vi "IMAQDevice.contents.vi"() -> ()   [LabVIEW 2014, in "IMAQDevice.lvlib"]
uses:
  IMAQDevice.lvlib
panel:
  out "error out":errorcluster
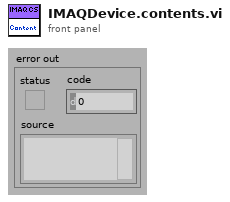
[diagram p1: front panel]
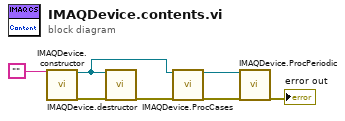
[diagram p0: block diagram]
diagram:
  n1 = call "IMAQDevice.constructor.vi"("name"="") -> ("i ref out"=w6:refnum<vi>, "error out"=w7:errorcluster)  [unwired: 16 in, 1 out]
  n2 = call "IMAQDevice.destructor.vi"("i ref in"=w6, "error in (no error)"=w7) -> ("error out"=w3:errorcluster)  [unwired: 17 in]
  n3 = call "IMAQDevice.ProcCases.vi"("i ref in"=w6, "error in (no error)"=w3) -> ("i ref out"=w5:refnum<vi>, "error out"=w4:errorcluster)  [unwired: 15 in, 1 out]
  n4 = call "IMAQDevice.ProcPeriodic.vi"("i ref in"=w5, "error in (no error)"=w4) -> ("error out"=→"error out":errorcluster)  [unwired: 15 in, 2 out]
